vi "make_q.vi"(8 "error in (no error)":errorcluster, 9 "Queue Data":T1, 10 "Command":string, 11 "name (unnamed)":string) -> (0 "error out":errorcluster, 3 "Queue out":refnum<queue>)   [LabVIEW 2020]
uses:
  Type Defs/Message.ctl
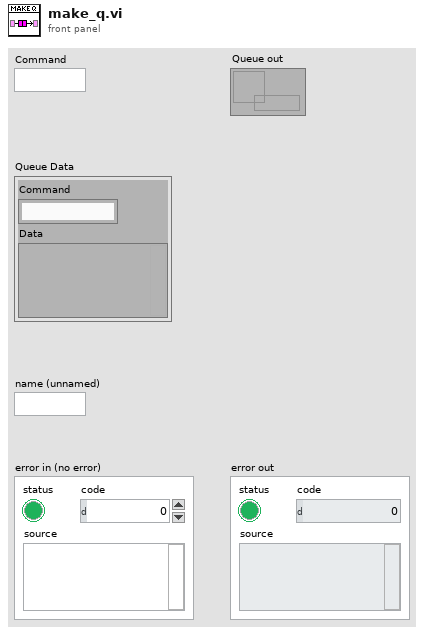
[diagram p1: front panel]
types:
  T1 = typedef "Message.ctl" = cluster{"Command":string, "Data":variant}
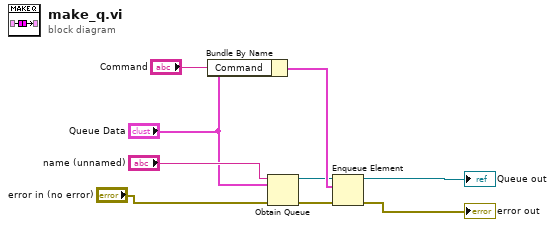
[diagram p0: block diagram]
diagram:
  n1 = Bundle By Name "Bundle By Name"(cluster="Queue Data", "Command"="Command") -> (w3:T1)
  n2 = Obtain Queue(name (unnamed)="name (unnamed)", element data type="Queue Data", error in (no error)="error in (no error)") -> (queue out=w2:refnum<queue>, error out=w4:errorcluster)  [unwired: 2 in, 1 out]
  n3 = Enqueue Element(queue=w2, element=w3, error in (no error)=w4) -> (queue out=→"Queue out":refnum<queue>, error out=→"error out":errorcluster)  [unwired: 1 in, 1 out]
